vi "solar Menu.vi"(7 "VIRef":refnum<vi>, 8 "error in (no error)":errorcluster, 9 "ItemTag":string, 10 "MenuRef":refnum<k9>, 11 "solar in":refnum<class "solar.lvclass">) -> (0 "error out":errorcluster, 3 "solar out":refnum<class "solar.lvclass">)   [LabVIEW 2018, in "solar.lvclass"]
doc: "This handles the target's menu selection."
uses:
  solar.lvclass
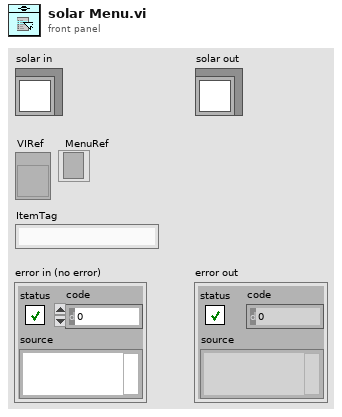
[diagram p1: front panel]
types:
  T1 = typedef "solar_ctl SOLAR Refnum.ctl" = refnum<k1>
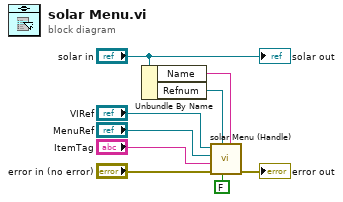
[diagram p0: block diagram]
diagram:
  n1 = Unbundle By Name("solar in") -> ("Name"=w2:string, "Refnum"=w1:T1)
  n2 = call "solar Menu (Handle).vi"("Target"=w2, "Is SOLAR UI? (F)"=FALSE, "SOLAR Refnum"=w1, "error in (no error)"="error in (no error)", "ItemTag"="ItemTag", "MenuRef"="MenuRef", "VIRef"="VIRef") -> ("error out"=→"error out":errorcluster)  [unwired: 4 in]
  "solar out" <- "solar in"
